vi "E727_StageSetup.vi"(8 "error in":errorcluster, 9 "StageRunningIn":bool, 10 "Position 2":dbl[](array[numeric]), 11 "StageOn/Off":bool) -> (0 "error out":errorcluster, 1 "StageChannels":string[](array[string]), 2 "Current position":dbl[](array[numeric]) format="%.6f", 3 "StageRunningOut":bool)   [LabVIEW 2022 SP3]
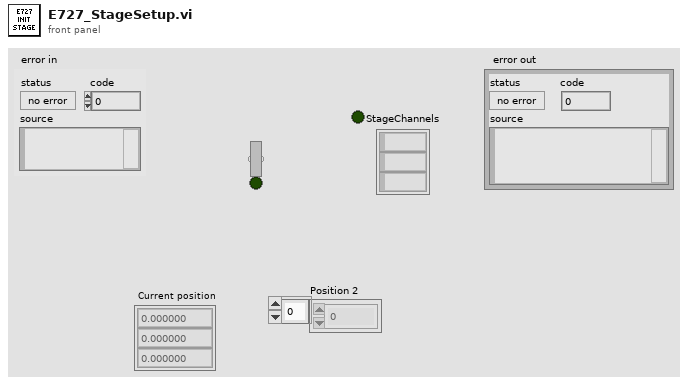
[diagram p1: front panel]
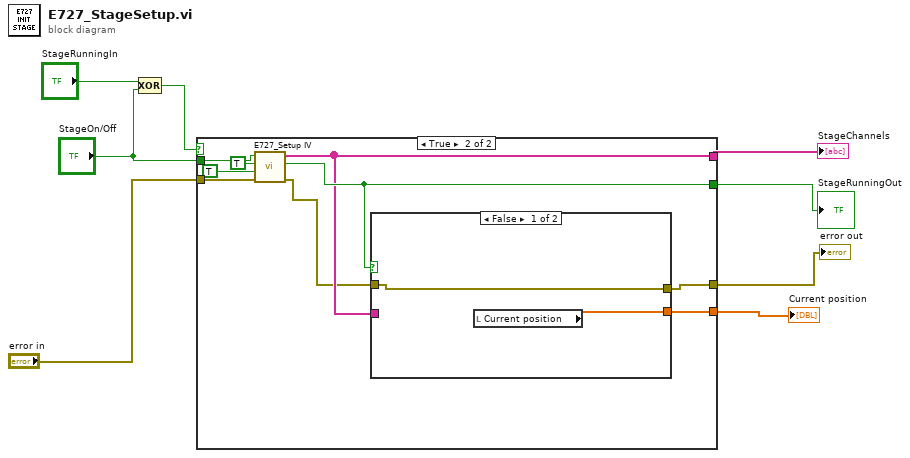
[diagram p0: block diagram]
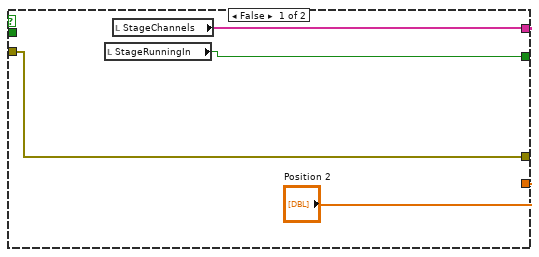
[diagram p2: hidden frame]
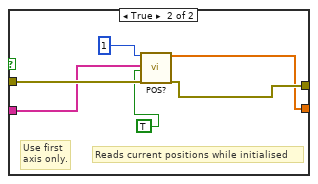
[diagram p3: hidden frame]
diagram:
  n1 = Compound Arithmetic op=XOR("StageRunningIn", "StageOn/Off") -> (w2:bool)
  n2 = case shown="True" w2 {
    tunnel: "StageOn/Off" -> [_ w21]
    tunnel: [w11 w19] -> w7
    tunnel: [w12 w18] -> w6
    tunnel: "error in" -> [w10 w20]
    tunnel: [w10 w16] -> w4
    tunnel: ["Position 2" w15] -> w3
    frame False {
      n3 = local read "StageRunningIn"() -> (w11:bool)
      n4 = local read "StageChannels"() -> (w12:string[])
    }
    frame True {
      n5 = call "E727_Setup IV.vi"("On/Off"=w21, "Move to middle?"=TRUE, "Perform autozero?"=TRUE, "error in"=w20) -> ("Conn. Axis"=w18:string[], "Running"=w19:bool, "error out"=w17:errorcluster)  [unwired: 4 in]
      n6 = case shown="False" w19 {
        tunnel: w18 -> [_ w24]
        tunnel: w17 -> [w23 w29]
        tunnel: [w23 w28] -> w16
        tunnel: [w22 w25] -> w15
        frame False {
          n7 = local read "Current position"() -> (w22:dbl[])
        }
        frame True {
          # "Reads current positions while initialised"
          # "Use first\naxis only."
          n8 = call "POS?.vi"("System no."=1, "Axes to query"=w24, "All axes?"=TRUE, "error in"=w29) -> ("Position"=w25:dbl[], "error out"=w28:errorcluster)  [unwired: 1 in, 13 out]
        }
      }
    }
  }
  "StageRunningOut" <- w7
  "StageChannels" <- w6
  "error out" <- w4
  "Current position" <- w3
